vi "initialise.vi"(8 "error in (no error)":errorcluster, 11 "DAQmxAnalogOut in":refnum<class "AnalogOutDL101207DAQmx.lvclass">) -> (0 "error out":errorcluster, 3 "DAQmxAnalogOut out":refnum<class "AnalogOutDL101207DAQmx.lvclass">)   [LabVIEW 2010, in "AnalogOutDL101207DAQmx.lvclass"]
doc: "The dynamic dispatch-version of this VI initalises the plug-in object by allocating and initalising any dynamic resources need."
uses:
  AnalogOutDL101207DAQmx.lvclass
  GenericAnalogOut/GenericAnalogOut/GenericAnalogOut.lvclass
  AnalogOutDL101207DAQmx.lvclass/AnalogOutDL101207DAQmx.ctl
  <vilib>/DAQmx/create/channels.llb/DAQmx Create Channel (AO-Voltage-Basic).vi
  common/classes/ErrorController/ErrorController/class_data.vi
  common/classes/ErrorController/ErrorController/ErrorController.lvclass
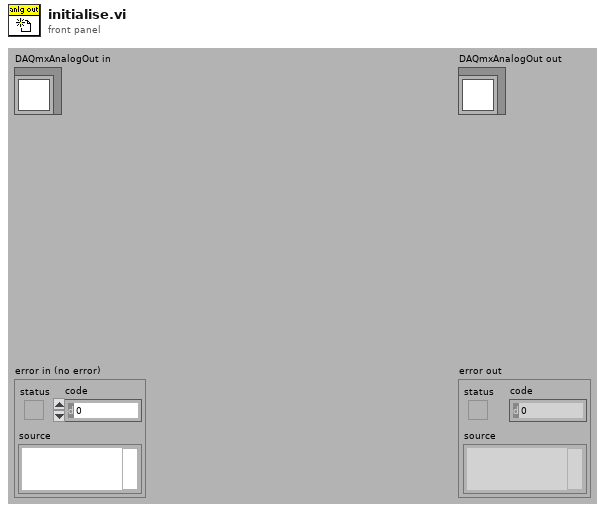
[diagram p1: front panel]
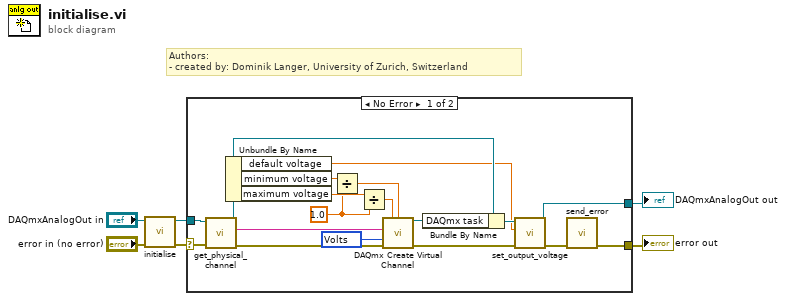
[diagram p0: block diagram]
diagram:
  # "Authors: \n- created by: Dominik Langer, University of Zurich, Switzerland"
  n1 = call-parent "initialise.vi"("error in (no error)"="error in (no error)", "GenericPlugin in"="DAQmxAnalogOut in") -> ("error out"=w4:errorcluster, "GenericPlugin out"=w3:refnum<class "AnalogOutDL101207DAQmx.lvclass">)  [unwired: 8 out]
  n2 = case shown="No Error" w4 {
    selector: w4 -> [w24 w25]
    tunnel: w3 -> [w23 w26]
    tunnel: [w10 w26] -> w2
    tunnel: [w7 w25] -> w1
    frame No Error {
      w18 = dbl[unit] 1.0 ("y")
      w15 = 10348 items=["Volts"=10348, "From Custom Scale"=10065] ("units")
      n3 = call "get_physical_channel.vi"("error in (no error)"=w24, "DAQmxAnalogOut in"=w23) -> ("error out"=w22:errorcluster, "DAQmx Physical Channel"=w21:tag, "DAQmxAnalogOut out"=w13:refnum<class "AnalogOutDL101207DAQmx.lvclass">)  [unwired: 7 out]
      n4 = Unbundle By Name(w13) -> ("default voltage"=w9:dbl[unit], "minimum voltage"=w20:dbl[unit], "maximum voltage"=w19:dbl[unit])
      n5 = Divide(x=w20, y=w18) -> (x/y=w16:dbl)
      n6 = Divide(x=w19, y=w18) -> (x/y=w17:dbl)
      n7 = call-poly <vilib>:"DAQmx Create Virtual Channel.vi"("maximum value"=w17, "minimum value"=w16, "physical channels"=w21, "units"=w15, "error in"=w22) -> ("task out"=w14:refnum<k21>, "error out"=w12:errorcluster)  [unwired: 4 in, 5 out]
      n8 = Bundle By Name(cluster=w13, "DAQmx task"=w14) -> (w11:refnum<class "AnalogOutDL101207DAQmx.lvclass">)
      n9 = call-dynamic "set_output_voltage.vi"("error in (no error)"=w12, "output value"=w9, "DAQmxAnalogOut in"=w11) -> ("error out"=w8:errorcluster, "DAQmxAnalogOut out"=w10:refnum<class "AnalogOutDL101207DAQmx.lvclass">)  [unwired: 7 in]
      n10 = call "send_error.vi"("error in (no error)"=w8) -> ("error out"=w7:errorcluster)  [unwired: 10 in]
    }
    frame Error {
    }
  }
  "error out" <- w1
  "DAQmxAnalogOut out" <- w2
